vi "step2 TestIfUpperLayerSolved.vi"(8 "error in (no error)":errorcluster, 11 "cube in":T1) -> (0 "error out":errorcluster, 2 "upper layer solved?":bool)   [LabVIEW 2011]
uses:
  Typedef/cube.ctl
  Typedef/face.ctl
  Typedef/cube rotate direction.ctl
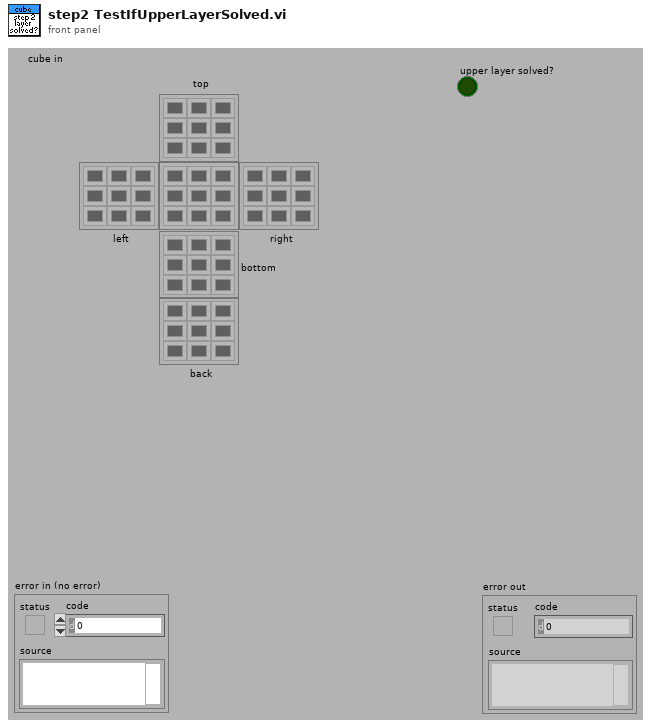
[diagram p1: front panel]
types:
  T1 = typedef "cube.ctl" = cluster{"top":T2, "left":T2, "right":T2, "bottom":T2, "back":T2, "front":T2}
  T2 = typedef "face.ctl" = u32[][]
  T3 = typedef "cube rotate direction.ctl" = enum16{"up", "down", "left", "right"}
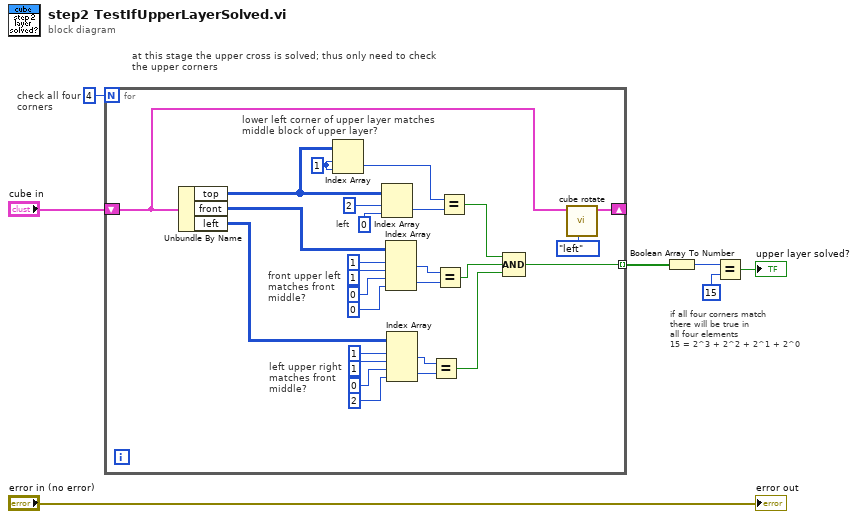
[diagram p0: block diagram]
diagram:
  # "check all four\ncorners"
  # "if all four corners match\nthere will be true in\nall four elements\n15 = 2^3 + 2^2 + 2^1 + 2^0"
  # "at this stage the upper cross is solved; thus only need to check\nthe upper corners"
  n1 = for {
    N: 4 -> [_]
    shift-right: [w8] -> _
    shift-left: "cube in" -> [w9]
    tunnel: [w10] -> w5 mode=indexing
    w30 = 1 ("index (row)")
    # "left upper right\nmatches front\nmiddle?"
    # "front upper left\nmatches front\nmiddle?"
    # "lower left corner of upper layer matches\nmiddle block of upper layer?"
    # "left"
    n2 = Unbundle By Name(w9) -> ("top"=w32:T2, "front"=w25:T2, "left"=w18:T2)
    n3 = Index Array(array=w32, index (row)=w30, index (col)=w30) -> (element=w34:u32)
    n4 = Index Array(array=w32, index (row)=2, index (col)=0 ("disabled index (col)")) -> (element=w31:u32)
    n5 = Index Array(array=w25, index (row) #1=1 ("index (row)"), index (col) #1=1 ("disabled index (col)"), index (row) #2=0 ("index (row)"), index (col) #2=0 ("disabled index (col)")) -> (element #1=w17:u32, element #2=w16:u32)
    n6 = Index Array(array=w18, index (row) #1=1 ("index (row)"), index (col) #1=1 ("disabled index (col)"), index (row) #2=0 ("index (row)"), index (col) #2=2 ("disabled index (col)")) -> (element #1=w15:u32, element #2=w14:u32)
    n7 = Equal?(x=w15, y=w14) -> (x = y?=w12:bool)
    n8 = Equal?(x=w17, y=w16) -> (x = y?=w13:bool)
    n9 = Equal?(x=w34, y=w31) -> (x = y?=w33:bool)
    n10 = Compound Arithmetic op=AND(w33, w13, w12) -> (w10:bool)
    n11 = call "cube rotate.vi"("cube rotation direction"=cube_rotate_direction."left", "cube in"=w9) -> ("cube out"=w8:T1)  [unwired: 8 in, 1 out]
  }
  n12 = Boolean Array To Number(Boolean array=w5) -> (number=w4:u32)
  n13 = Equal?(x=w4, y=u32 15) -> (x = y?=→"upper layer solved?":bool)
  "error out" <- "error in (no error)"
